vi "EJERCICIO 1 DE LOGICA COMBINACIONAL.vi"() -> ()   [LabVIEW 2013]
panel:
  out "SALIDA":bool
  in  "D":bool
  in  "C":bool
  in  "B":bool
  in  "A":bool
  # "universidad de cundinamarca \n    ingenieria de sistemas\n    andy leandro camargo\n            electiva pro IV"
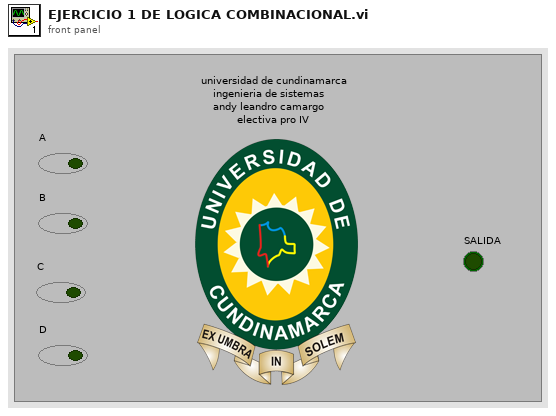
[diagram p1: front panel]
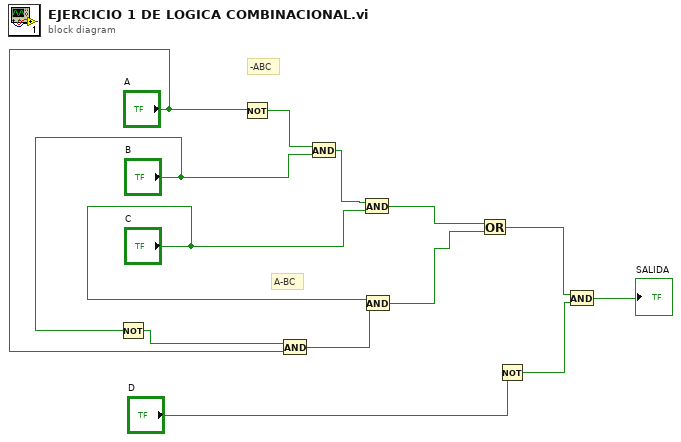
[diagram p0: block diagram]
diagram:
  # "A-BC"
  # "-ABC"
  n1 = Not(x="B") -> (.not. x?=w8:bool)
  n2 = Not(x="A") -> (.not. x?=w12:bool)
  n3 = And(x=w8, y="A") -> (x .and. y?=w6:bool)
  n4 = And(x=w12, y="B") -> (x .and. y?=w11:bool)
  n5 = And(x=w11, y="C") -> (x .and. y?=w5:bool)
  n6 = And(x="C", y=w6) -> (x .and. y?=w4:bool)
  n7 = Or(x=w5, y=w4) -> (x .or. y?=w2:bool)
  n8 = Not(x="D") -> (.not. x?=w3:bool)
  n9 = And(x=w2, y=w3) -> (x .and. y?=→"SALIDA":bool)
